vi "FFT1D(CuLab_vs_LabVIEW).vi"() -> ()   [LabVIEW 2020]
doc: "This benchmark is designed to demonstrate execution performance improvement when executing FFT and IFFT operations on a GPU."
uses:
  956bade7-a26b-4376-82d1-4f43b9b25d0c.vi
  a45b64e6-426e-4566-b00d-58499d731ec9.vi
  2d4acfdf-3b2f-4360-8aac-546d4cc334b7.vi
  e3d6266a-341e-462f-8124-2d714a455819.vi
  <vilib>/Utility/High Resolution Relative Seconds.vi
  <vilib>/Ngene/CuLab - GPU Accelerated Toolkit/Toolkit/Low_Level/Tensor_Classes/T_Children/T1D/T1D_Children/T1D_SGL/Push.vi
  <vilib>/Ngene/CuLab - GPU Accelerated Toolkit/Toolkit/API/Signal Processing/Transforms/CU_FFT/T1D/CU_FFT_T1D_R2C.vi
  <vilib>/Analysis/2dsp.llb/Real FFT.vi
  <vilib>/Ngene/CuLab - GPU Accelerated Toolkit/Toolkit/API/Numeric/Absolute/T1D/CU_Absolute_T1D_CSG.vi
  <vilib>/Ngene/CuLab - GPU Accelerated Toolkit/Toolkit/Low_Level/Tensor_Classes/T_Children/T1D/T1D_Children/T1D_SGL/Create_Push.vi
  <vilib>/Ngene/CuLab - GPU Accelerated Toolkit/Toolkit/Low_Level/Tensor_Classes/T_Children/T1D/T1D_Children/T1D_SGL/Pull.vi
  <vilib>/Analysis/NI_AALBase.lvlib
  <vilib>/Ngene/CuLab - GPU Accelerated Toolkit/Toolkit/CuLab.lvlib
  <vilib>/Analysis/NI_AALPro.lvlib
  <vilib>/Ngene/CuLab - GPU Accelerated Toolkit/Toolkit/Low_Level/Tensor_Classes/T_Children/T1D/T1D_Children/T1D_SGL/T1D_SGL.lvclass
panel:
  out "Improvement":dbl[](array[numeric])=[36.50360161856616, 36.185390325613305, 32.351256610011, 23.08342449593315, 18.012349103850973, 12.973898855180295, 11.137741951849097, 8.067769605828097, 5.418153632890173, 3.7918215982069228, 1.639118464616597, 0.7101025180299668, 0.38249590933755945, 0.1783960621707361] format="%.2f"
  out "Iteration":i32=9
  out "FFT_Size":i32=1024
  out "Computing on":string="CPU"
  out "GPU Model":string="NVIDIA GeForce GTX 1650 Ti"
  out "CPU Model":string="Intel(R) Core(TM) i7-10750H CPU @ 2.60GHz  "
  in  "No. of Repetitions":i32=10
  in  "FFT Size Stop (2^N)":i32=23
  in  "FFT Size Start (2^N)":i32=10
  out "FFT Sizes":i32[](array[numeric])=[8388608, 4194304, 2097152, 1048576, 524288, 262144, 131072, 65536, 32768, 16384, 8192, 4096, 2048, 1024] format="%.2p"
  out "Performance Improvement":cluster{i32[], dbl[]}(graph)={[8388608, 4194304, 2097152, 1048576, 524288, 262144, 131072, 65536, 32768, 16384, 8192, 4096, 2048, 1024], [36.50360161856616, 36.185390325613305, 32.351256610011, 23.08342449593315, 18.012349103850973, 12.973898855180295, 11.137741951849097, 8.067769605828097, 5.418153632890173, 3.7918215982069228, 1.639118464616597, 0.7101025180299668, 0.38249590933755945, 0.1783960621707361]}
  out "Execution Times":cluster{i32[], "FFT mean Exec Time":dbl[]}[](graph)=[{[8388608, 4194304, 2097152, 1048576, 524288, 262144, 131072, 65536, 32768, 16384, 8192, 4096, 2048, 1024], "FFT mean Exec Time"=[0.5604835999984061, 0.263929000000644, 0.11997139999948558, 0.04432710000037332, 0.01939929999934975, 0.00795300000027055, 0.00345269999888842, 0.0015119000017875805, 0.0006983999992371537, 0.0003060000017285347, 0.00011900000026798807, 4.850000186706893e-05, 2.359999780310318e-05, 1.089999932446517e-05]}, {[8388608, 4194304, 2097152, 1048576, 524288, 262144, 131072, 65536, 32768, 16384, 8192, 4096, 2048, 1024], "FFT mean Exec Time"=[0.015354200000729179, 0.0072938000012072735, 0.003708399999595713, 0.001920299997436814, 0.0010770000008051284, 0.0006130000001576263, 0.0003099999994446989, 0.00018739999723038636, 0.00012889999925391749, 8.069999967119657e-05, 7.259999983943999e-05, 6.829999983892776e-05, 6.170000051497482e-05, 6.10999995842576e-05]}]
  # "Overview: 1D FFT Benchmark.\nRequirements: PC with Nvidia GPU, with latest version of GPU driver and CuLab Toolkit installed.\nInstructions:\n1. Run the VI with the current benchmarking parameters.\n2. Wait for the completion of the execution. \nNote: It might take some time to perform the computations.\n3. Observe the timing and speedup results on the graphs."
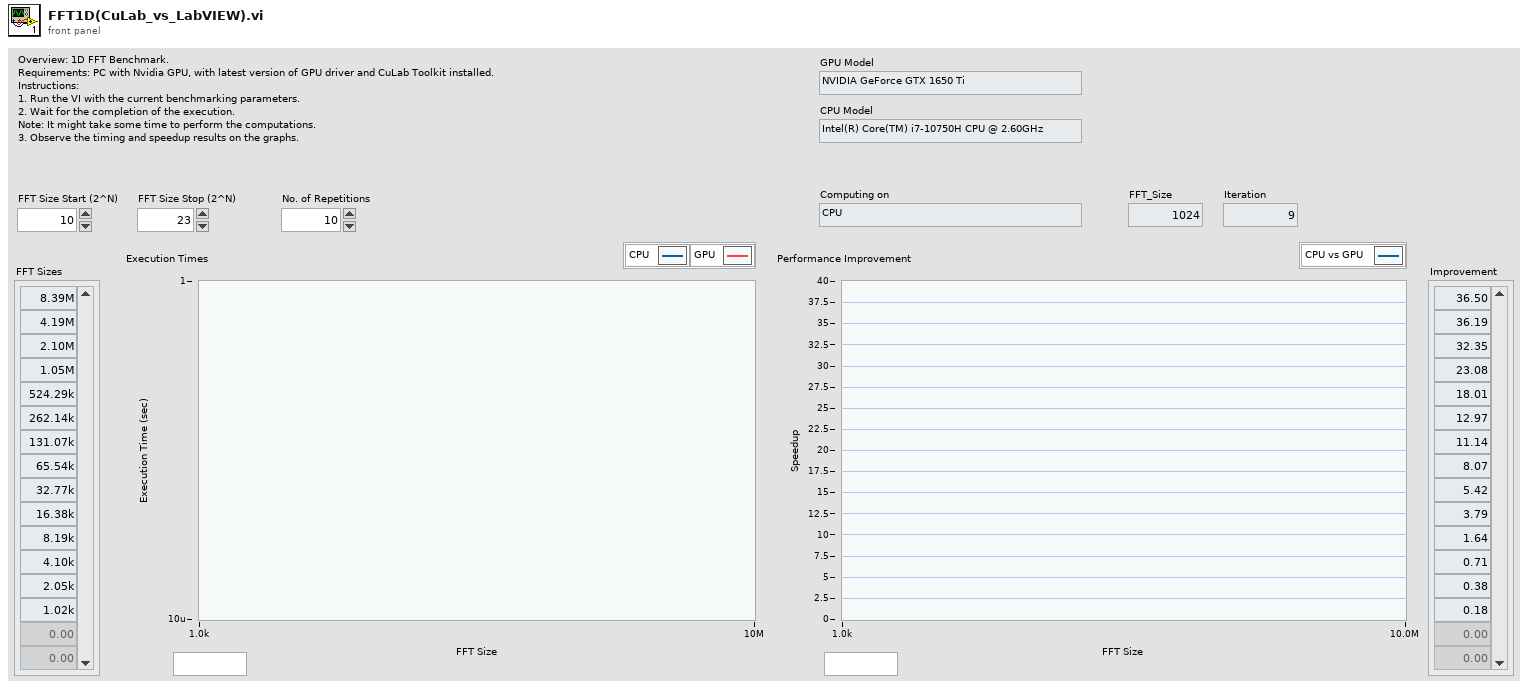
[diagram p1: front panel]
types:
  T1 = typedef "CuLab.lvlib/Properties.ctl" = cluster{"Index":i32, "Name":string}
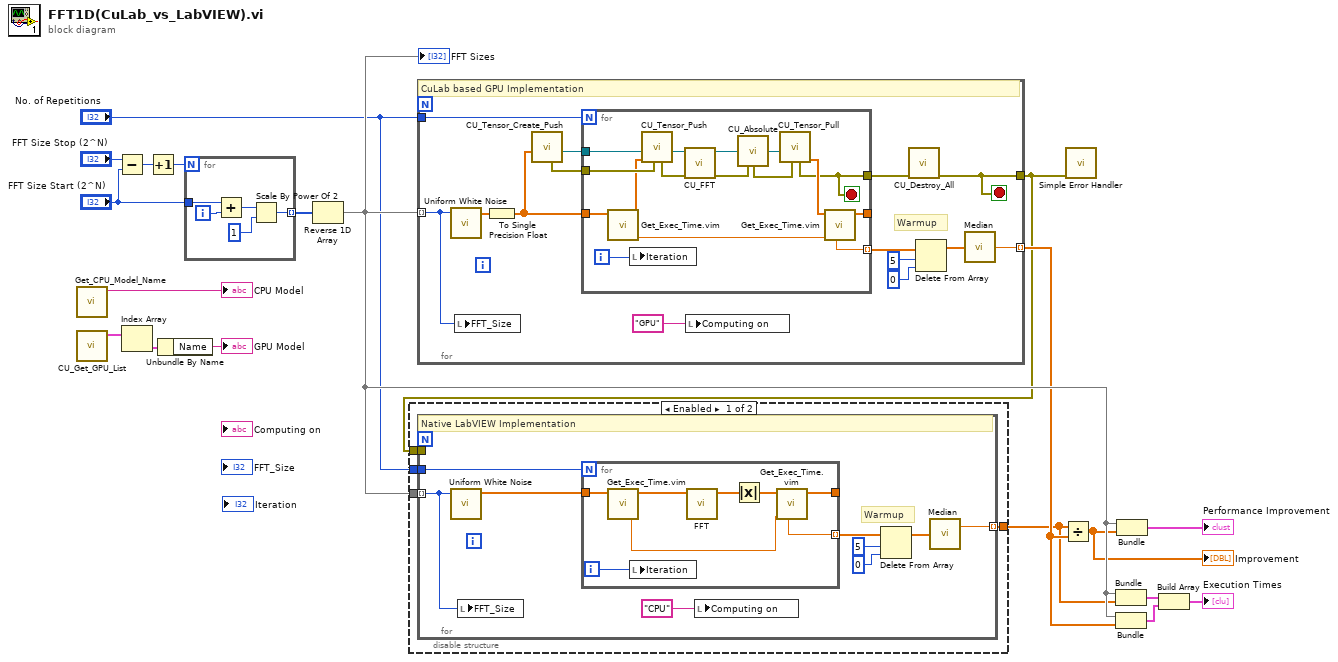
[diagram p0: block diagram]
diagram:
  n1 = call "Get_CPU_Model_Name.vi"() -> ("CPU Model"=→"CPU Model":string)  [unwired: 11 in]
  n2 = call <vilib>:"CU_Get_GPU_List.vi"() -> ("Devices"=w9:T1[])  [unwired: 10 in, 1 out]
  n3 = Subtract(x="FFT Size Stop (2^N)", y="FFT Size Start (2^N)") -> (x-y=w17:i32)
  n4 = Index Array(array=w9) -> (element=w8:T1)  [unwired: 1 in]
  n5 = Increment(x=w17) -> (x+1=w16:i32)
  n6 = Unbundle By Name(w8) -> ("Name"=→"GPU Model":string)
  n7 = for {
    N: w16 -> [_]
    tunnel: "FFT Size Start (2^N)" -> [w24]
    tunnel: [w20] -> w12 mode=indexing
    i -> [w23]
    n8 = Add(x=w24, y=w23) -> (x+y=w22:i32)
    n9 = Scale By Power Of 2(n=w22, x=1) -> (x*2^n=w20:i32)
  }
  n10 = Reverse 1D Array(array=w12) -> (reversed array=w19:i32[])
  "FFT Sizes" <- w19
  n11 = for {
    tunnel: [w27] -> w11
    tunnel: [w36] -> w13 mode=indexing
    tunnel: w19 -> [w25] mode=indexing
    tunnel: "No. of Repetitions" -> [w32]
    stop <- w27 stop-if-true
    # "Warmup"
    # "CuLab based GPU Implementation"
    n12 = call <vilib>:"Uniform White Noise.vi"("samples"=w25) -> ("uniform white noise"=w28:dbl[])  [unwired: 9 in, 1 out]
    n13 = local write "FFT_Size"(w25) -> ()
    n14 = To Single Precision Float(number=w28) -> (single precision float=w29:sgl[])
    n15 = call-poly <vilib>:"CU_Tensor_Create_Push.vi"("CPU_Data_1D_SGL"=w29) -> ("T1D_SGL out"=w38:refnum<class "T1D_SGL.lvclass">, "error out"=w37:errorcluster)  [unwired: 9 in]
    n16 = for {
      N: w32 -> [_]
      tunnel: w38 -> [w51]
      tunnel: w37 -> [w48]
      tunnel: [w41] -> w31
      tunnel: [w52] -> w30 mode=indexing
      tunnel: w29 -> [w47]
      tunnel: [w44] -> _
      i -> [w49]
      stop <- w41 stop-if-true
      n17 = call "Get_Exec_Time.vim"("error in (no error)"=w47) -> ("T(n)"=w53:dbl, "error out"=w46:sgl[])  [unwired: 6 in, 1 out]
      n18 = local write "Iteration"(w49) -> ()
      n19 = call-poly <vilib>:"CU_Tensor_Push.vi"("error in (no error)"=w48, "CPU_Data_1D_SGL"=w46, "T1D_SGL in"=w51) -> ("T1D_SGL out"=w50:refnum<class "T1D_SGL.lvclass">, "error out"=w54:errorcluster)  [unwired: 7 in]
      n20 = call-poly <vilib>:"CU_FFT.vi"("error in"=w54, "X"=w50) -> ("error out"=w40:errorcluster, "FFT {X}"=w43:refnum<class "T1D_CSG.lvclass">)  [unwired: 8 in]
      n21 = call-poly <vilib>:"CU_Absolute.vi"("x"=w43, "error in (no error)"=w40) -> ("Dest out"=w42:refnum<class "T1D_SGL.lvclass">, "error out"=w39:errorcluster)  [unwired: 12 in]
      n22 = call-poly <vilib>:"CU_Tensor_Pull.vi"("error in (no error)"=w39, "T1D_SGL in"=w42) -> ("Dest out"=w45:sgl[], "error out"=w41:errorcluster)  [unwired: 7 in, 1 out]
      n23 = call "Get_Exec_Time.vim"("T(n-1)"=w53, "error in (no error)"=w45) -> ("error out"=w44:sgl[], "dT"=w52:dbl)  [unwired: 5 in, 1 out]
    }
    n24 = local write "Computing on"("GPU" ("Info")) -> ()
    n25 = call <vilib>:"CU_Destroy_All.vi"("error in"=w31) -> ("error out"=w27:errorcluster)  [unwired: 10 in]
    n26 = Delete From Array(array=w30, length=5, index=0) -> (array with subset deleted=w35:dbl[])  [unwired: 1 out]
    n27 = call <vilib>:"Median.vi"("X"=w35) -> ("median"=w36:dbl)  [unwired: 1 out]
  }
  n28 = disable-structure shown="Enabled" {
    disable-tunnel: "No. of Repetitions" -> [w58 _]
    disable-tunnel: w11 -> [w57 _]
    disable-tunnel: [w56 _] -> w4
    disable-tunnel: w19 -> [w55 _]
    frame Enabled {
      n29 = for {
        tunnel: [w63] -> w56 mode=indexing
        tunnel: w55 -> [w59] mode=indexing
        tunnel: w58 -> [w62]
        tunnel: w57 -> [_]
        # "Warmup"
        # "Native LabVIEW Implementation"
        n30 = call <vilib>:"Uniform White Noise.vi"("samples"=w59) -> ("uniform white noise"=w61:dbl[])  [unwired: 9 in, 1 out]
        n31 = local write "FFT_Size"(w59) -> ()
        n32 = for {
          N: w62 -> [_]
          tunnel: w61 -> [w74]
          tunnel: [w72] -> _
          tunnel: [w70] -> w67 mode=indexing
          i -> [w69]
          n33 = call "Get_Exec_Time.vim"("error in (no error)"=w74) -> ("T(n)"=w71:dbl, "error out"=w73:dbl[])  [unwired: 6 in, 1 out]
          n34 = local write "Iteration"(w69) -> ()
          n35 = call-poly <vilib>:"FFT.vi"("X"=w73) -> ("FFT {X}"=w75:cdb[])  [unwired: 9 in, 1 out]
          n36 = Absolute Value(x=w75) -> (abs(x)=w68:dbl[])
          n37 = call "Get_Exec_Time.vim"("T(n-1)"=w71, "error in (no error)"=w68) -> ("error out"=w72:dbl[], "dT"=w70:dbl)  [unwired: 5 in, 1 out]
        }
        n38 = local write "Computing on"("CPU" ("Info")) -> ()
        n39 = Delete From Array(array=w67, length=5, index=0) -> (array with subset deleted=w64:dbl[])  [unwired: 1 out]
        n40 = call <vilib>:"Median.vi"("X"=w64) -> ("median"=w63:dbl)  [unwired: 1 out]
      }
    }
    frame Disabled {
    }
  }
  n41 = Divide(x=w4, y=w13) -> (x/y=w1:dbl[])
  "Improvement" <- w1
  n42 = call <vilib>:"Simple Error Handler.vi"("error in (no error)"=w11) -> ()  [unwired: 4 in, 5 out]
  n43 = Bundle(w19, w4) -> (w6:cluster{i32[], dbl[]})  [unwired: 1 in]
  n44 = Bundle(w19, w13) -> (w5:cluster{i32[], dbl[]})  [unwired: 1 in]
  n45 = Bundle(w19, w1) -> (→"Performance Improvement":cluster{i32[], dbl[]})  [unwired: 1 in]
  n46 = Build Array(w6, w5) -> (→"Execution Times":cluster{i32[], dbl[]}[])
